vi "Open VI Server Application Control.vi"(6 "open block diagram (F)":bool, 7 "open front panel (F)":bool, 8 "error in (no error)":errorcluster, 10 "run VI (F)":bool, 11 "VI refnum":refnum<vi>) -> (0 "error out":errorcluster)   [LabVIEW 2011]
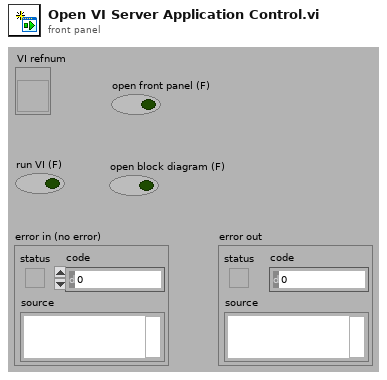
[diagram p1: front panel]
types:
  T1 = enum32{"Bad", "Idle", "Run top level", "Running"}
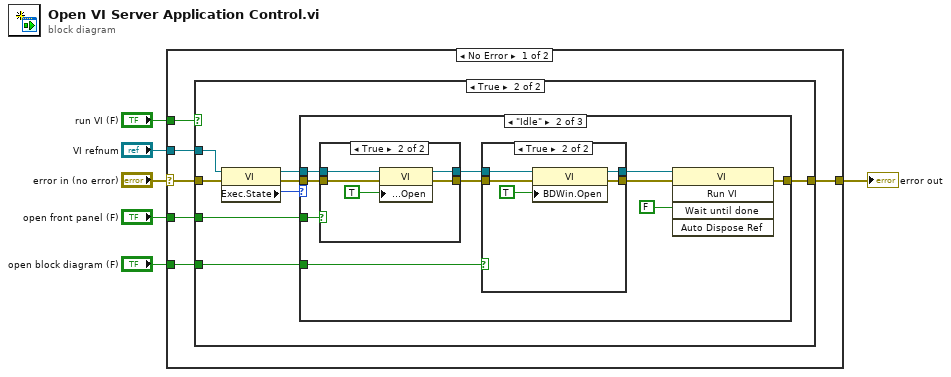
[diagram p0: block diagram]
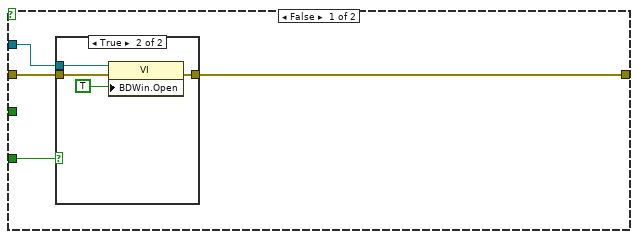
[diagram p2: hidden frame]
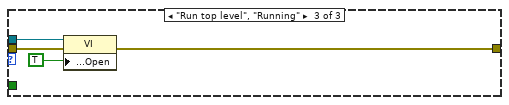
[diagram p7: hidden frame]
diagram:
  n1 = case shown="No Error" "error in (no error)" {
    selector: "error in (no error)" -> [w7 w59]
    tunnel: "VI refnum" -> [w12 _]
    tunnel: "run VI (F)" -> [w11 _]
    tunnel: "open front panel (F)" -> [w10 _]
    tunnel: "open block diagram (F)" -> [w9 _]
    tunnel: [w8 w59] -> w2
    frame No Error {
      n2 = case shown="True" w11 {
        tunnel: w12 -> [w16 w26]
        tunnel: w10 -> [_ w25]
        tunnel: w9 -> [w15 w24]
        tunnel: w7 -> [w14 w23]
        tunnel: [w13 w22] -> w8
        frame False {
          n3 = case shown="True" w15 {
            tunnel: w16 -> [_ w20]
            tunnel: w14 -> [w17 w19]
            tunnel: [w17 w18] -> w13
            frame False {
            }
            frame True {
              n4 = property class="VI"(reference=w20, error in=w19, "BDWin.Open"=TRUE ("Front Panel Window:Open")) -> (error out=w18:errorcluster)  [unwired: 1 out]
            }
          }
        }
        frame True {
          n5 = property class="VI"(reference=w26, error in=w23) -> (reference out=w29:refnum<vi>, error out=w28:errorcluster, "Exec.State"=w27:T1)
          n6 = case shown="\"Idle\"" w27 {
            tunnel: w28 -> [w30 w34 w56]
            tunnel: w29 -> [_ w40 w58]
            tunnel: w25 -> [_ w38 _]
            tunnel: w24 -> [_ w35 _]
            tunnel: [w30 w31 w55] -> w22
            frame "Bad", Default {
            }
            frame "Idle" {
              n7 = case shown="True" w38 {
                tunnel: w40 -> [w49 w53]
                tunnel: [w49 w52] -> w37
                tunnel: w34 -> [w48 w51]
                tunnel: [w48 w50] -> w33
                frame False {
                }
                frame True {
                  n8 = property class="VI"(reference=w53, error in=w51, "Front Panel.Open"=TRUE ("Front Panel Window:Open")) -> (reference out=w52:refnum<vi>, error out=w50:errorcluster)
                }
              }
              n9 = case shown="True" w35 {
                tunnel: w37 -> [w42 w46]
                tunnel: [w42 w45] -> w36
                tunnel: w33 -> [w41 w44]
                tunnel: [w41 w43] -> w32
                frame False {
                }
                frame True {
                  n10 = property class="VI"(reference=w46, error in=w44, "BDWin.Open"=TRUE ("Front Panel Window:Open")) -> (reference out=w45:refnum<vi>, error out=w43:errorcluster)
                }
              }
              n11 = invoke class="VI" method="Run VI"(reference=w36, error in=w32, "Wait until done"=FALSE ("Wait Until Done")) -> (error out=w31:errorcluster)  [unwired: 2 in, 4 out]
            }
            frame "Run top level", "Running" {
              n12 = property class="VI"(reference=w58, error in=w56, "Front Panel.Open"=TRUE ("Front Panel Window:Open")) -> (error out=w55:errorcluster)  [unwired: 1 out]
            }
          }
        }
      }
    }
    frame Error {
    }
  }
  "error out" <- w2
